vi "1B Spoof Reality.vi"(10 "Wind Direction":dbl, 11 "Wind Speed":dbl=1.0) -> (0 "Apparent Wind\nDirection":T3, 1 "Apparent Wind\nSpeed":T2, 2 "Robot velocity":T1, 3 "Robot\nHeading":T4 format="%05.1f", 4 "Boat Path":cluster{"X Position":dbl, "Y Position":dbl}[](array[cluster]), 5 "Robot UTM Location":T5, 6 "XY Graph":cluster{dbl, dbl}[](graph))   [LabVIEW 2011]
uses:
  2-RIO/2 Typedefs/UTM Location.ctl
  2-RIO/2 Typedefs/heading.ctl
  2-RIO/2 Typedefs/apparent wind direction.ctl
  2-RIO/2 Typedefs/apparent wind speed.ctl
  2-RIO/2 Typedefs/Velocity.ctl
  2-RIO/2 Globals/2 Global.vi
panel:
  out "Absolute Wind":cluster{"East":dbl, "North":dbl}
  out "Velocity internal":dbl[](array[numeric])
  out "Speed":dbl
  # "This is the Bass. It's catchy. You like it."
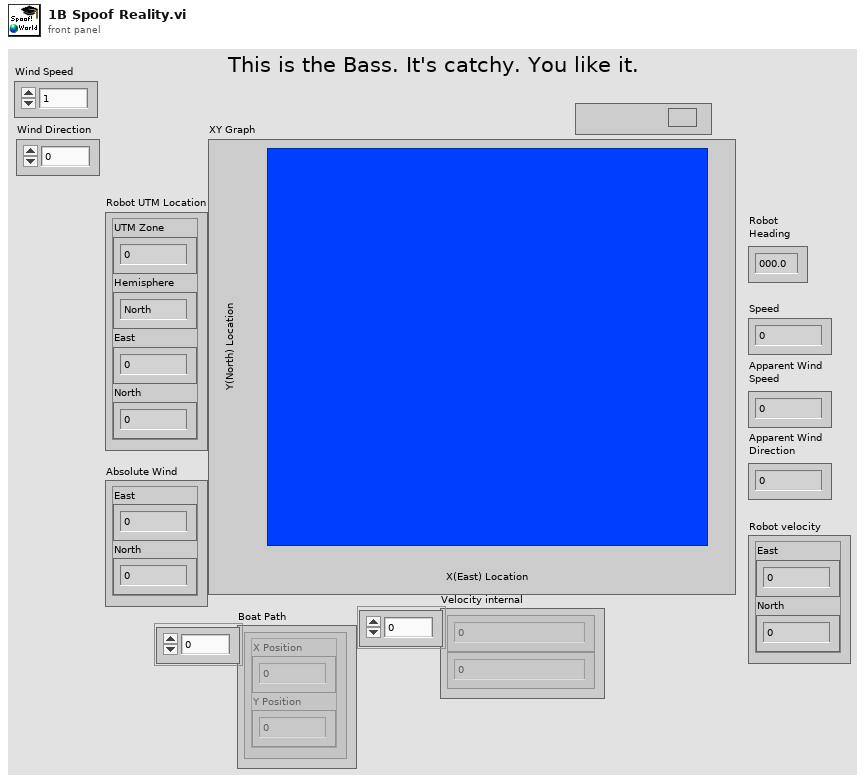
[diagram p1: front panel]
types:
  T1 = typedef "Velocity.ctl" = cluster{"East":dbl, "North":dbl}
  T2 = typedef "apparent wind speed.ctl" = dbl
  T3 = typedef "apparent wind direction.ctl" = dbl
  T4 = typedef "heading.ctl" = dbl
  T5 = typedef "UTM Location.ctl" = cluster{"UTM Zone":dbl, "Hemisphere":enum16{"North", "South"}, "East":dbl, "North":dbl}
  T6 = typedef "setpoints to boat.ctl" = cluster{"Sail Position":T7, "Rudder Angle":T8}
  T7 = typedef "sail setpt.ctl" = dbl
  T8 = typedef "rudder angle.ctl" = dbl
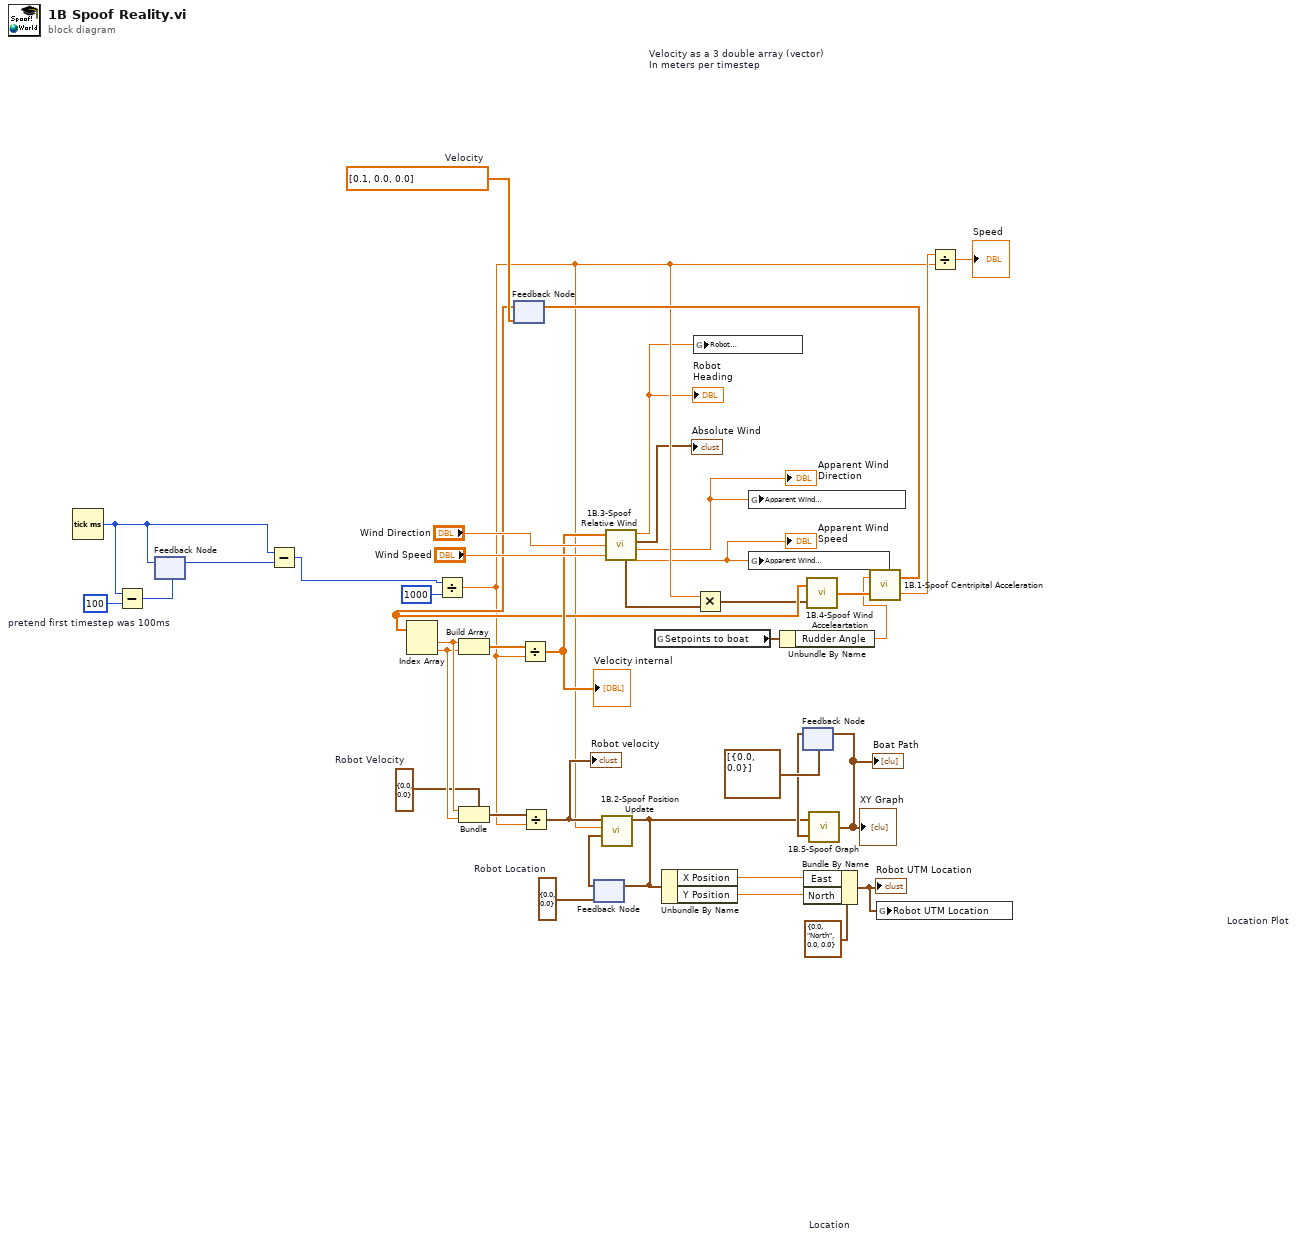
[diagram p0: block diagram]
diagram:
  w1 = u32 100  # pretend first timestep was 100ms
  w13 = T1 {"East"=0.0, "North"=0.0}  # Robot Velocity
  w31 = dbl[] [0.1, 0.0, 0.0]  # Velocity
  w38 = cluster{"X Position":dbl, "Y Position":dbl} {"X Position"=0.0, "Y Position"=0.0}  # Robot Location
  n1 = Tick Count (ms)() -> (millisecond timer value=w2:u32)
  n2 = Subtract(x=w2, y=w1) -> (x-y=w3:u32)
  n3 = feedback #1(w3) -> (w5:u32)
  n4 = feedback-in #1(w2) -> ()
  n5 = Subtract(x=w2, y=w5) -> (x-y=w4:u32)
  n6 = Divide(x=w4, y=u32 1000 ("x")) -> (x/y=w20:dbl)
  n7 = feedback #2 "Velocity as a 3 double array (vector)\nIn meters per timestep"(w31) -> (w23:dbl[])
  n8 = Index Array(array=w23) -> (element #1=w28:dbl, element #2=w27:dbl)  [unwired: 2 in]
  n9 = Build Array(w28, w27) -> (w26:dbl[])
  n10 = Bundle(cluster=w13, "East"=w28, "North"=w27) -> (w30:T1)
  n11 = Divide(x=w26, y=w20) -> (x/y=w25:dbl[])
  "Velocity internal" <- w25
  n12 = Divide(x=w30, y=w20) -> (x/y=w24:T1)
  "Robot velocity" <- w24
  n13 = feedback #3 "Location"(w38) -> (w37:cluster{"X Position":dbl, "Y Position":dbl})
  n14 = call "1B.2-Spoof Position Update.vi"("Old Position"=w37, "dt"=w20, "Robot Velocity"=w24) -> ("New Position"=w19:cluster{"X Position":dbl, "Y Position":dbl})  [unwired: 8 in]
  n15 = feedback-in #3(w19) -> ()
  n16 = call "1B.3-Spoof Relative Wind.vi"("Wind Speed"="Wind Speed", "Wind Angle"="Wind Direction", "Velocity (3 array)"=w25) -> ("Apparent Wind\nSpeed"=w8:T2, "Perceived Wind"=w9:cluster{"X Position":dbl, "Y Position":dbl}, "Apparent Wind\nDirection"=w7:T3, "Global Wind"=→"Absolute Wind":cluster{"X Position":dbl, "Y Position":dbl}, "Robot\nHeading"=w10:T4)  [unwired: 1 in]
  "Robot\nHeading" <- w10
  "Apparent Wind\nDirection" <- w7
  "Apparent Wind\nSpeed" <- w8
  n17 = global read "2 Global.vi" "Setpoints to boat"() -> (w12:T6)
  n18 = Unbundle By Name(w19) -> ("X Position"=w17:dbl, "Y Position"=w16:dbl)
  n19 = global write "2 Global.vi" "Robot\nHeading"(w10) -> ()
  n20 = Multiply(x=w20, y=w9) -> (x*y=w21:cluster{"X Position":dbl, "Y Position":dbl})
  n21 = global write "2 Global.vi" "Apparent Wind\nDirection"(w7) -> ()
  n22 = global write "2 Global.vi" "Apparent Wind\nSpeed"(w8) -> ()
  n23 = Unbundle By Name(w12) -> ("Rudder Angle"=w11:T8)
  n24 = feedback #4 "Location Plot"(cluster{dbl, dbl}[] [{0.0, 0.0}] ("XY Graph")) -> (w34:cluster{dbl, dbl}[])
  n25 = Bundle By Name(cluster=T5 {"UTM Zone"=0.0, "Hemisphere"=enum."North", "East"=0.0, "North"=0.0} ("Robot UTM Location 2"), "East"=w17, "North"=w16) -> (w15:T5)
  "Robot UTM Location" <- w15
  n26 = call "1B.4-Spoof Wind Acceleartation.vi"("Perceived Wind"=w21, "Old Velocity"=w23) -> ("New Velocity"=w22:dbl[])
  n27 = call "1B.5-Spoof Graph.vi"("XY Graph"=w34, "New Position"=w19) -> ("Array"=w35:cluster{"X Position":dbl, "Y Position":dbl}[])
  "XY Graph" <- w35
  "Boat Path" <- w35
  n28 = feedback-in #4(w35) -> ()
  n29 = call "1B.1-Spoof Centripital Acceleration.vi"("Old Velocity"=w22, "Rudder Angle"=w11) -> ("Speed"=w29:dbl, "New Velocity"=w33:dbl[])
  n30 = feedback-in #2(w33) -> ()
  n31 = global write "2 Global.vi" "Robot UTM Location"(w15) -> ()
  n32 = Divide(x=w29, y=w20) -> (x/y=→"Speed":dbl)
